vi "VF Device Ramp Up.vi"(8 "error in":errorcluster, 11 "Island in":refnum<class "Island.lvclass">) -> (0 "error out":errorcluster, 3 "Island out":refnum<class "Island.lvclass">)   [LabVIEW 2018, in "Island Actor.lvlib" / "Island.lvclass"]
uses:
  Island.lvclass
  C:/Users/Administrator/Desktop/2018LabVIEW EMS/EMS Generic Actor/EMS Generic/EMS Generic.lvclass
  C:/Users/Administrator/Desktop/2018LabVIEW EMS/Device Communication and Control Abstract Actor/Device Communication and Control Abstract/Device Communication and Control Abstract.lvclass
  <vilib>/ORNL/CSEISMIC DDS/CSEISMIC DDS Base/Data Types/DER_SetPointP.ctl
  <vilib>/ORNL/CSEISMIC DDS/CSEISMIC DDS Base/Data Types/Controls/DeviceID.ctl
  <vilib>/ActorFramework/Actor/Actor.lvclass/Actor.ctl
  Device Communication and Control Abstract Actor/Device Communication and Control Abstract/Device Communication and Control Abstract.lvclass/Device Communication and Control Abstract.ctl
  Device Communication and Control Abstract Actor/Device Communication and Control Abstract Messages/Set DER SetPointP Msg/Set DER SetPointP Msg.lvclass/Set DER SetPointP Msg.ctl
  <vilib>/ActorFramework/Message Enqueuer/Message Enqueuer.lvclass/Message Enqueuer.ctl
  Device Communication and Control Abstract Actor/Device Communication and Control Abstract Messages/Set DER SetPointP Msg/Send Set DER SetPointP.vi
  <vilib>/ActorFramework/Actor/Read Caller Enqueuer.vi
  <vilib>/ActorFramework/Message Enqueuer/Enqueue.vi
  Device Communication and Control Abstract Actor/Device Communication and Control Abstract/Device Communication and Control Abstract.lvclass
  C:/Program Files (x86)/National Instruments/LabVIEW 2018/vi.lib/ActorFramework/Actor/Actor.lvclass
  Device Communication and Control Abstract Actor/Device Communication and Control Abstract Messages/Set DER SetPointP Msg/Set DER SetPointP Msg.lvclass
  C:/Program Files (x86)/National Instruments/LabVIEW 2018/vi.lib/ActorFramework/Message/Message.lvclass
  <vilib>/ActorFramework/Message Priority Queue/Priority Enqueue.vi
  <vilib>/ORNL/CSEISMIC DDS/CSEISMIC DDS Base/CSEISMIC DDS.lvclass
  EMS Generic Actor/EMS Generic/EMS Generic.lvclass
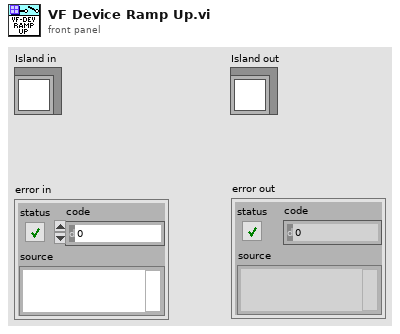
[diagram p1: front panel]
types:
  T1 = typedef "CSEISMIC DDS.lvlib/CSEISMIC DDS.lvclass/DER_SetPointP.ctl" = cluster{"DeviceID":T2, "RealPower (kW)":dbl[]}
  T2 = typedef "CSEISMIC DDS.lvlib/CSEISMIC DDS.lvclass/DeviceID.ctl" = string
  T3 = typedef "CSEISMIC DDS.lvlib/CSEISMIC DDS.lvclass/IED_Status.ctl" = cluster{"DeviceID":T2, "Timestamp":T4, "MicrogridID":u8, "Active":bool, "Inactive":bool, "Error":i32, "Fault":bool, "ErrorString":string}
  T4 = typedef "CSEISMIC DDS.lvlib/CSEISMIC DDS.lvclass/Timestamp.ctl" = cluster{"Seconds":u64, "Remainder":u64}
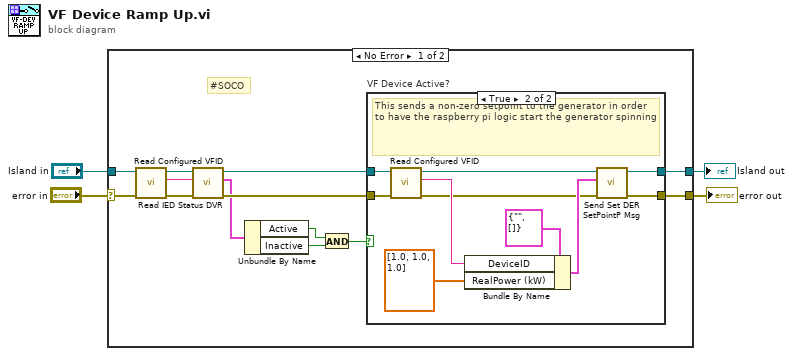
[diagram p0: block diagram]
diagram:
  n1 = case shown="No Error" "error in" {
    selector: "error in" -> [w11 w30]
    tunnel: [w17 w31] -> w4
    tunnel: "Island in" -> [w16 w31]
    tunnel: [w9 w30] -> w1
    frame No Error {
      # "#SOCO"
      n2 = call "Read Configured VFID.vi"("error in"=w11, "EMS Generic in"=w16) -> ("error out"=w12:errorcluster, "VFID"=w13:T2, "EMS Generic out"=w15:refnum<class "Island.lvclass">)  [unwired: 7 in]
      n3 = call "Read IED Status DVR.vi"("error in"=w12, "DeviceID"=w13, "EMS Generic in"=w15) -> ("error out"=w10:errorcluster, "IED_Status"=w8:T3, "EMS Generic out"=w14:refnum<class "Island.lvclass">)  [unwired: 5 in, 1 out]
      n4 = Unbundle By Name(w8) -> ("Active"=w6:bool, "Inactive"=w7:bool)
      n5 = And(x=w6, y=w7) -> (x .and. y?=w5:bool)
      n6 = case "VF Device Active?" shown="True" w5 {
        tunnel: [w19 w29] -> w17
        tunnel: w14 -> [w19 w24]
        tunnel: w10 -> [w18 w23]
        tunnel: [w18 w25] -> w9
        frame False {
        }
        frame True {
          # "This sends a non-zero setpoint to the generator in order to have the raspberry pi logic start the generator spinning"
          n7 = call "Read Configured VFID.vi"("error in"=w23, "EMS Generic in"=w24) -> ("error out"=w20:errorcluster, "VFID"=w22:T2, "EMS Generic out"=w21:refnum<class "Island.lvclass">)  [unwired: 7 in]
          n8 = Bundle By Name(cluster=T1 {"DeviceID"="", "RealPower (kW)"=[]} ("DER_SetPointP"), "DeviceID"=w22, "RealPower (kW)"=dbl[] [1.0, 1.0, 1.0]) -> (w26:T1)
          n9 = call "Send Set DER SetPointP Msg.vi"("error in"=w20, "DER_SetPointP"=w26, "SCADA Sub Abstract in"=w21) -> ("error out"=w25:errorcluster, "SCADA Sub Abstract out"=w29:refnum<class "Island.lvclass">)  [unwired: 7 in]
        }
      }
    }
    frame Error {
    }
  }
  "Island out" <- w4
  "error out" <- w1
